vi "Validate.vi"(8 "error in (no error)":errorcluster, 11 "Action Interface in":refnum<class>) -> (0 "error out":errorcluster, 1 "Valid?":bool, 3 "Action Interface out":refnum<class>)   [LabVIEW 2019, in "ProjectBuilder.lvlib" / "Project Action.lvclass"]
doc: "Call Validate_Do.vi if the class type uses the interface. If the interface is not used 'Valid?' will be set to false."
uses:
  Class/Project Action/Project Action.lvclass
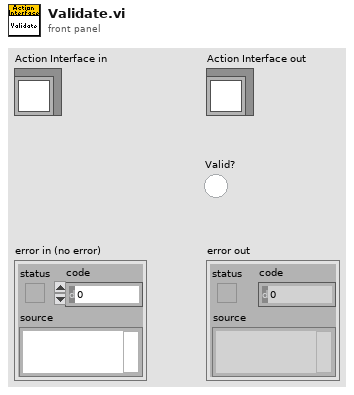
[diagram p1: front panel]
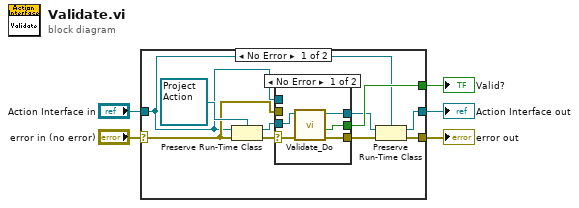
[diagram p0: block diagram]
diagram:
  n1 = case shown="No Error" "error in (no error)" {
    selector: "error in (no error)" -> [w10 w24]
    tunnel: [w9 w24] -> w4
    tunnel: [w7 w23] -> w2
    tunnel: "Action Interface in" -> [w6 w23]
    tunnel: [w14 _] -> w1
    frame No Error {
      n2 = Preserve Run-Time Class(object in=w6, error in=w10, 2:refnum<class "Project Action.lvclass"> refnum ("ProjectBuilder.lvlib:Project Action Interface.lvclass")) -> (object out=w12:refnum<class "Project Action.lvclass">, error out=w13:errorcluster)
      n3 = case shown="No Error" w13 {
        selector: w13 -> [w17 _]
        tunnel: [w20 w22] -> w15
        tunnel: [w19 w21] -> w8
        tunnel: [w18 _] -> w14
        tunnel: w12 -> [w16 _]
        tunnel: w10 -> [_ w22]
        tunnel: w6 -> [_ w21]
        frame No Error {
          n4 = call-dynamic "Validate_Do.vi"("error in (no error)"=w17, "Action in"=w16) -> ("error out"=w20:errorcluster, "Valid?"=w18:bool, "Action out"=w19:refnum<class "Project Action.lvclass">)  [unwired: 7 in]
        }
        frame Error {
        }
      }
      n5 = Preserve Run-Time Class(object in=w8, error in=w15, 2:w6) -> (object out=w7:refnum<class>, error out=w9:errorcluster)
    }
    frame Error {
    }
  }
  "error out" <- w4
  "Action Interface out" <- w2
  "Valid?" <- w1
